vi "setEdgeTrigger.vi"(7 "Source":string, 8 "error in (no error)":errorcluster, 9 "Edge":T1, 10 "Threshold [V]":dbl, 11 "ScopeKeysight in":refnum<class "ScopeKeysight.lvclass">) -> (0 "error out":errorcluster, 3 "ScopeKeysight out":refnum<class "ScopeKeysight.lvclass">)   [LabVIEW 2023, in "ScopeKeysight.lvclass"]
doc: "<b>Author:</b> Wolfgang\n<b>Description:</b> Configure Edge Trigger."
uses:
  ScopeKeysight.lvclass
  Data/scopeEdgeTrigger.ctl
  ScopeKeysight.lvclass/ScopeKeysight.ctl
  Driver/Public/Configure/Trigger/Configure Trigger (Edge).vi
  Driver/Keysight-DSQx3014T.lvlib
  sweScope.lvlib
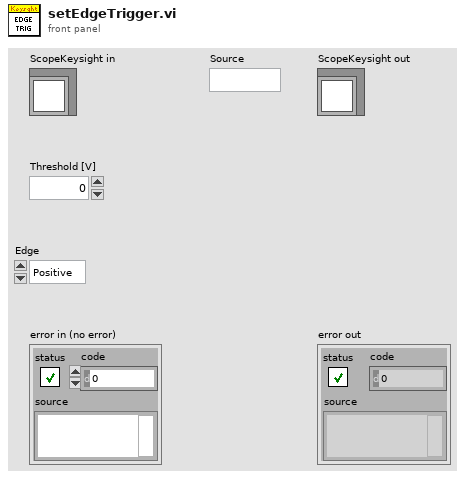
[diagram p1: front panel]
types:
  T1 = typedef "sweScope.lvlib/scopeEdgeTrigger.ctl" = enum16{"Positive", "Negative", "Either"}
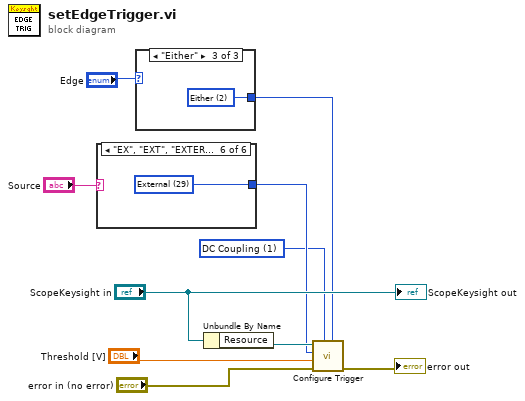
[diagram p0: block diagram]
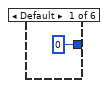
[diagram p2: hidden frame]
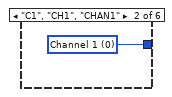
[diagram p3: hidden frame]
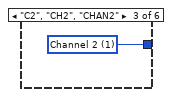
[diagram p4: hidden frame]
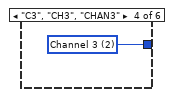
[diagram p5: hidden frame]
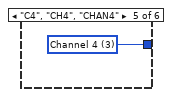
[diagram p6: hidden frame]
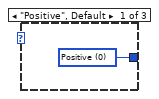
[diagram p7: hidden frame]
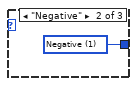
[diagram p8: hidden frame]
diagram:
  w1 = 1 items=["AC Coupling", "DC Coupling", "Low Frequency Reject"] ("Input Coupling (0: AC Coupling)")
  n1 = case shown="\"EX\", \"EXT\", \"EXTERNAL\"" "Source" {
    tunnel: [0 ("Channel Name (0: Channel 1)") w12 w13 w14 w15 w16] -> w4
    frame Default {
    }
    frame "C1", "CH1", "CHAN1" {
      w12 = 0 items=["Channel 1", "Channel 2", "Channel 3", "Channel 4"] ("Channel Name (0: Channel 1)")
    }
    frame "C2", "CH2", "CHAN2" {
      w13 = 1 items=["Channel 1", "Channel 2", "Channel 3", "Channel 4"] ("Channel Name (0: Channel 1)")
    }
    frame "C3", "CH3", "CHAN3" {
      w14 = 2 items=["Channel 1", "Channel 2", "Channel 3", "Channel 4"] ("Channel Name (0: Channel 1)")
    }
    frame "C4", "CH4", "CHAN4" {
      w15 = 3 items=["Channel 1", "Channel 2", "Channel 3", "Channel 4"] ("Channel Name (0: Channel 1)")
    }
    frame "EX", "EXT", "EXTERNAL" {
      w16 = 29 items=["Channel 1"=0, "Channel 2"=1, "Channel 3"=2, "Channel 4"=3, "D0"=13, "D1"=14, "D2"=15, "D3"=16, "D4"=17, "D5"=18, "D6"=19, "D7"=20, "D8"=21, "D9"=22, "D10"=23, "D11"=24, "D12"=25, "D13"=26, "D14"=27, "D15"=28, "External"=29, "Power Line"=30, "Waveform Generator"=31] ("Trigger Source (0: Channel 1)")
    }
  }
  n2 = case shown="\"Either\"" "Edge" {
    tunnel: [w17 w18 w19] -> w3
    frame "Positive", Default {
      w17 = 0 items=["Positive", "Negative", "Either", "Alternate"] ("Edge Slope (0: Positive)")
    }
    frame "Negative" {
      w18 = 1 items=["Positive", "Negative", "Either", "Alternate"] ("Edge Slope (0: Positive)")
    }
    frame "Either" {
      w19 = 2 items=["Positive", "Negative", "Either", "Alternate"] ("Edge Slope (0: Positive)")
    }
  }
  n3 = Unbundle By Name("ScopeKeysight in") -> ("Resource"=w8:refnum<visa-resource-name>)
  n4 = call-poly "Configure Trigger.vi"("Edge Slope (0: Positive)"=w3, "Input Coupling (0: AC Coupling)"=w1, "error in (no error)"="error in (no error)", "Trigger Level (0 V)"="Threshold [V]", "Trigger Source (0: Channel 1)"=w4, "VISA resource name"=w8) -> ("error out"=→"error out":errorcluster)  [unwired: 4 in, 1 out]
  "ScopeKeysight out" <- "ScopeKeysight in"
